vi "DLP2Recipe_XML_Write.vi"(8 "error in (no error)":errorcluster, 10 "data":T1, 11 "Recipe XML File Path":path) -> (0 "error out":errorcluster, 3 "XML File Path (duplicate)":path)   [LabVIEW 2022 SP3]
uses:
  Controls/DLP2RecipeV2.ctl
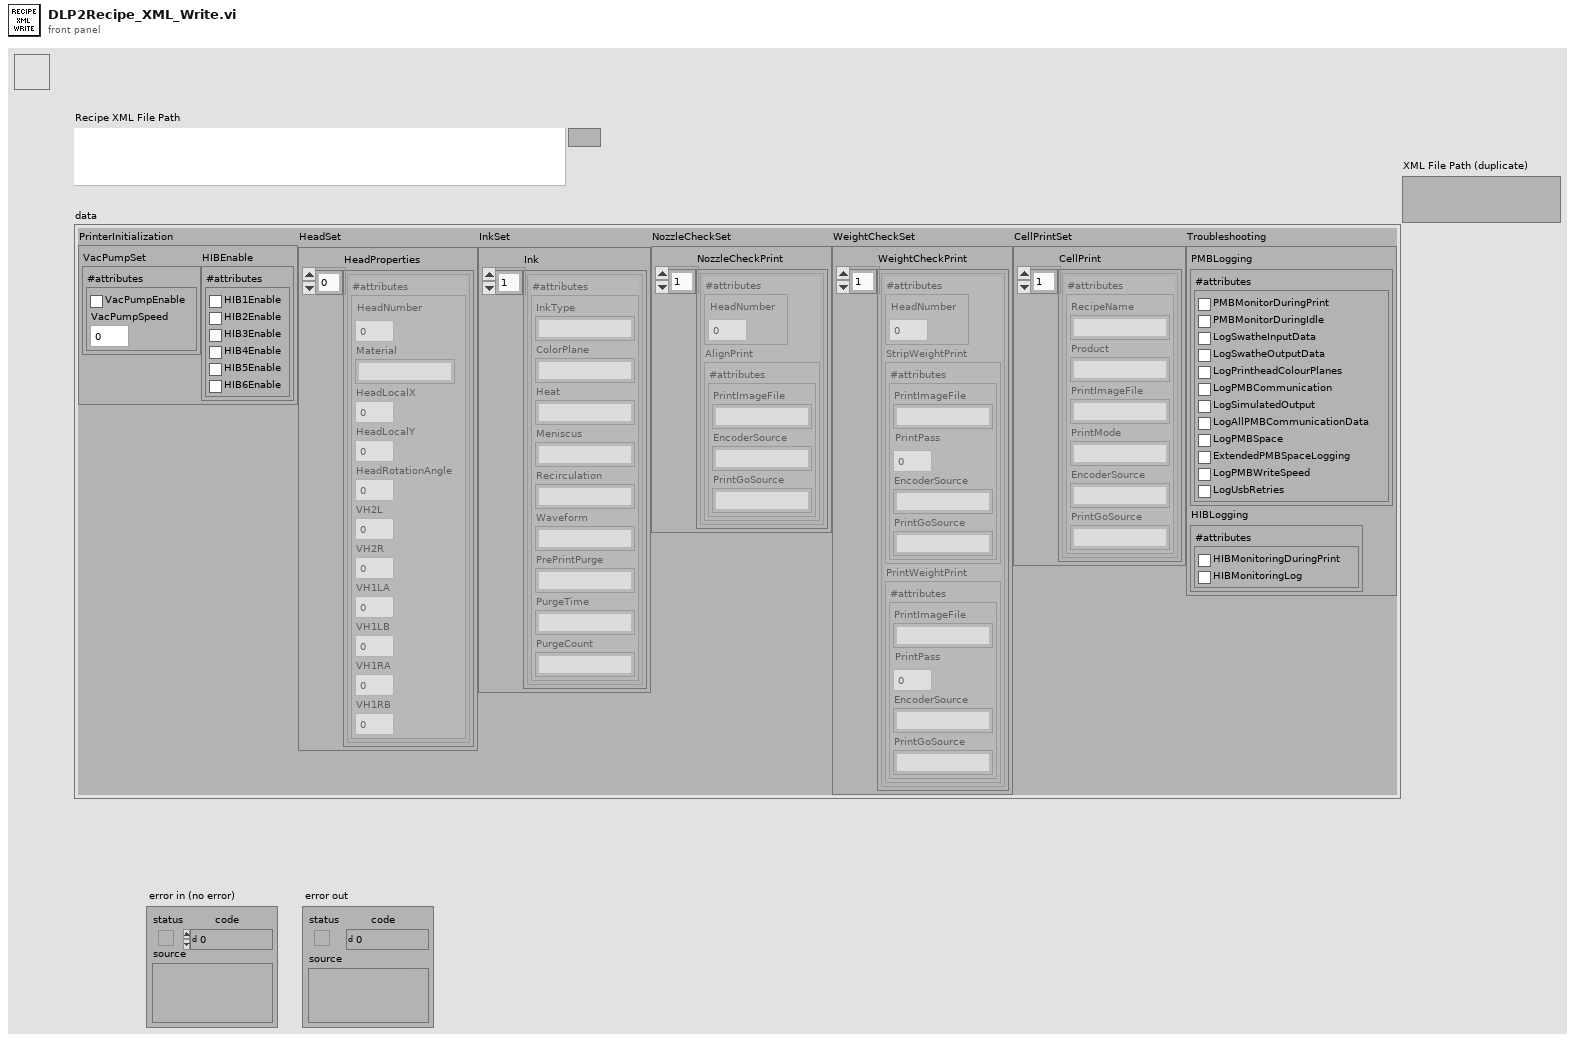
[diagram p1: front panel]
types:
  T1 = typedef "DLP2RecipeV2.ctl" = cluster{"PrinterInitialization":cluster{"VacPumpSet":cluster{"#attributes":cluster{"VacPumpEnable":bool, "VacPumpSpeed":dbl}}, "HIBEnable":cluster{"#attributes":cluster{"HIB1Enable":bool, "HIB2Enable":bool, "HIB3Enable":bool, "HIB4Enable":bool, "HIB5Enable":bool, "HIB6Enable":bool}}}, "HeadSet":cluster{"HeadProperties":cluster{"#attributes":cluster{"HeadNumber":u8, "Material":string, "HeadLocalX":dbl, "HeadLocalY":dbl, "HeadRotationAngle":dbl, "VH2L":dbl, "VH2R":dbl, "VH1LA":dbl, "VH1LB":dbl, "VH1RA":dbl, "VH1RB":dbl}}[]}, "InkSet":cluster{"Ink":cluster{"#attributes":cluster{"InkType":string, "ColorPlane":string, "Heat":string, "Meniscus":string, "Recirculation":string, "Waveform":string, "PrePrintPurge":string, "PurgeTime":string, "PurgeCount":string}}[]}, "NozzleCheckSet":cluster{"NozzleCheckPrint":cluster{"#attributes":cluster{"HeadNumber":u8}, "AlignPrint":cluster{"#attributes":cluster{"PrintImageFile":string, "EncoderSource":string, "PrintGoSource":string}}}[]}, "WeightCheckSet":cluster{"WeightCheckPrint":cluster{"#attributes":cluster{"HeadNumber":u8}, "StripWeightPrint":cluster{"#attributes":cluster{"PrintImageFile":string, "PrintPass":u8, "EncoderSource":string, "PrintGoSource":string}}, "PrintWeightPrint":cluster{"#attributes":cluster{"PrintImageFile":string, "PrintPass":u8, "EncoderSource":string, "PrintGoSource":string}}}[]}, "CellPrintSet":cluster{"CellPrint":cluster{"#attributes":cluster{"RecipeName":string, "Product":string, "PrintImageFile":string, "PrintMode":string, "EncoderSource":string, "PrintGoSource":string}}[]}, "Troubleshooting":cluster{"PMBLogging":cluster{"#attributes":cluster{"PMBMonitorDuringPrint":bool, "PMBMonitorDuringIdle":bool, "LogSwatheInputData":bool, "LogSwatheOutputData":bool, "LogPrintheadColourPlanes":bool, "LogPMBCommunication":bool, "LogSimulatedOutput":bool, "LogAllPMBCommunicationData":bool, "LogPMBSpace":bool, "ExtendedPMBSpaceLogging":bool, "LogPMBWriteSpeed":bool, "LogUsbRetries":bool}}, "HIBLogging":cluster{"#attributes":cluster{"HIBMonitoringDuringPrint":bool, "HIBMonitoringLog":bool}}}}
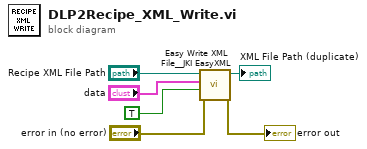
[diagram p0: block diagram]
diagram:
  n1 = call <vilib>:"Easy Write XML File__JKI EasyXML.vi"("error in (no error)"="error in (no error)", "Overwrite File? (false)"=TRUE, "LabVIEW Data"="data", "XML File Path"="Recipe XML File Path") -> ("error out"=→"error out":errorcluster, "XML File Path (duplicate)"=→"XML File Path (duplicate)":path)  [unwired: 6 in]
